vi "create_labview_ui_with_json_string.vi"(0 "json string":string, 11 "error in (no error)":errorcluster) -> (15 "error out":errorcluster)   [LabVIEW 2020]
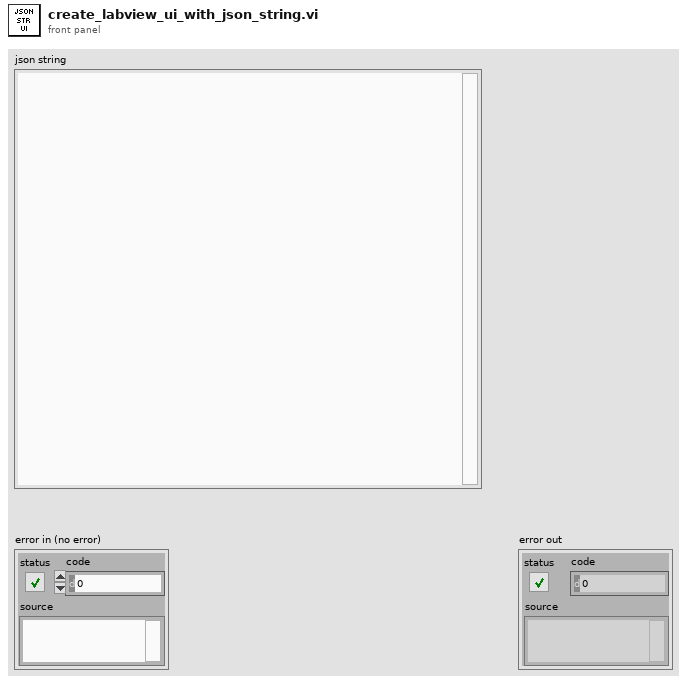
[diagram p1: front panel]
types:
  T1 = typedef "LVBoundsTypeDef.ctl" = cluster{"Width":u32, "Height":u32}
  T2 = typedef "LVPointTypeDef.ctl" = cluster{"Horizontal":i16, "Vertical":i16}
  T3 = typedef "LVPositionTypeDef.ctl" = cluster{"Left":i32, "Top":i32}
  T4 = cluster{"ViSize":cluster{"Width":i16, "Height":i16}, "ui elements":cluster{"io":string, "type":string, "bounds":T1, "location":T2, "label":cluster{"text":string, "label visible?":bool, "label position":T3, "label size":T1, "font size":u32}}[]}
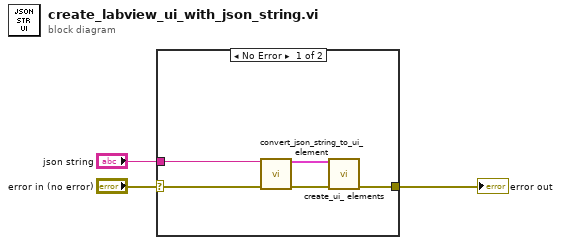
[diagram p0: block diagram]
diagram:
  n1 = case shown="No Error" "error in (no error)" {
    selector: "error in (no error)" -> [w7 w9]
    tunnel: [w5 w9] -> w2
    tunnel: "json string" -> [w4 _]
    frame No Error {
      n2 = call "convert_json_string_to_ui_element.vi"("json string"=w4, "error in (no error)"=w7) -> ("labview structure"=w8:T4, "error out"=w6:errorcluster)  [unwired: 12 in]
      n3 = call "create_ui_ elements.vi"("labview structure"=w8, "error in (no error)"=w6) -> ("error out"=w5:errorcluster)  [unwired: 13 in]
    }
    frame Error {
    }
  }
  "error out" <- w2
